vi "test Upload I32 C5-E.vi"(11 "Test Case In":refnum<class "Tests SDO Manager.lvclass">) -> (0 "error out":errorcluster, 3 "Test Case Out":refnum<class "Tests SDO Manager.lvclass">)   [LabVIEW 2020, in "Tests SDO Manager.lvclass"]
uses:
  Tests SDO Manager.lvclass
  C:/Program Files/National Instruments/LabVIEW 2026/vi.lib/Astemes/LUnit/Test Case.lvclass
  source/Logging/Logger/Logger.lvclass
  C:/Program Files/National Instruments/LabVIEW 2026/vi.lib/ActorFramework/Actor/Actor.lvclass
  HAL/HAL-Devices/source/PCAN USB Dongle/PCAN Basic 4/Configure Strategies/Read-Write CAN Frame Strategy/PCAN Basic4 Read-Write CAN CC Frame Strategy.lvclass
  D:/git/HAL/Source/Interfaces/IApplyConfiguration/IApplyConfiguration.lvclass
  HAL/Source/Communicator/Communicator.lvclass
  D:/git/HAL/Source/Interfaces/ICommunicate/ICommunicate.lvclass
  source/Logging/Logger/Logger.lvclass/Logger.ctl
  source/SDO Manager/SDO Manager/SDO Manager/SDO Manager.lvclass/SDO Manager.ctl
  <vilib>/ActorFramework/Message Enqueuer/Message Enqueuer.lvclass/Message Enqueuer.ctl
  <vilib>/Astemes/LUnit/Test Case.lvclass/Test Case.ctl
  <vilib>/ActorFramework/Stop Msg/Stop Msg.lvclass
  C:/Program Files/National Instruments/LabVIEW 2026/vi.lib/ActorFramework/Message/Message.lvclass
  HAL/Source/Interfaces/IMessage/IMessage.lvclass
  Tests SDO Manager.lvclass/Tests SDO Manager.ctl
  D:/git/HAL/HAL-Devices/source/PCAN USB Dongle/PCAN Basic 4/Configure Strategies/Base Configure Strategy/PCAN Basic4 Base Configure Strategy.lvclass
  D:/git/HAL/Source/Interfaces/IClose/IClose.lvclass
  D:/git/HAL/Source/Interfaces/IInitialize/IInitialize.lvclass
  D:/git/HAL/Source/Interfaces/IRunnable/IRunnable.lvclass
  D:/git/HAL/Source/Interfaces/IValidate Configuration/IValidate Configuration.lvclass
  D:/git/HAL/HAL-Devices/source/PCAN USB Dongle/PCAN Basic 4/Configure Strategies/Read-Write CAN Frame Strategy/PCAN Basic4 Read-Write CAN CC Frame Strategy.lvclass
  D:/git/HAL/Source/Interfaces/IInstrument/IInstrument.lvclass
  D:/git/HAL/Source/Communicator/Communicator.lvclass
  D:/git/HAL/Source/Interfaces/IConfigurable/IConfigurable.lvclass
  D:/git/CANopen-LabVIEW/source/Logging/Logger/Logger.lvclass
  4993e8ee-a06a-463a-9684-69129f64d5ce.vi
  source/SDO Manager/SDO Manager/SDO Manager/SDO Manager.lvclass
  source/Logging/Log Level.vi
  source/Logging/CANopen Logging.lvlib
  <vilib>/ActorFramework/Actor/Actor.lvclass
  source/SDO Manager/SDO Manager/SDO Manager/Upload I32.vi
  source/SDO Manager/SDO Manager/SDO Transfer/SDO abort code.ctl
  source/SDO Manager/SDO Manager/SDO Transfer/SDO Transfer.lvclass
  source/Typedefs/SDO Result.ctl
panel:
  out "SDO Result":T1={"Success"=FALSE, "SDO abort code"={"Null"=TRUE, "Value"=84082688}, "Data"={"Null"=TRUE, "Data"=[]}} {"SDO abort code"."Value" items=["Toggle bit not allowed"=84082688, "SDO protocol timed out"=84148224, "Client/server command specifier not valid or unknown"=84148225, "Invalid block size (block mode only)"=84148226, "Invalid sequence number (block mode only)"=84148227, "CRC error (block mode only)"=84148228, "Out of memory"=84148229, "Attempt to read a write only object"=100728833, "Attempt to write a read only object"=100728834, "Object does not exist in the object dictionary"=100794368, "Object cannot be mapped to the PDO"=100925505, "The number and length of the objects to be mapped would exceed PDO length"=100925506, "General parameter incompatibility reason"=100925507, "General internal incompatibility in the device"=100925511, "Access failed due to an hardware error"=101056512, "Data type does not match, length of service parameter does not match"=101122064, "Data type does not match, length of service parameter too high"=101122066, "Data type does not match, length of service parameter too low"=101122067, "Sub-index does not exist"=101253137, "Invalid value for parameter (download only)"=101253168, "Value of parameter written too high (download only)"=101253169, "Value of parameter written too low (download only)"=101253170, "Maximum value is less than minimum value"=101253174, "Resource not available: SDO connection"=101318691, "General error"=134217728, "Data cannot be transferred or stored to the application"=134217760, "Data cannot be transferred or stored to the application because of local control"=134217761, "Data cannot be transferred or stored to the application because of the present device stable"=134217762, "Object dictionary dynamic generation fails or no object dictionary is present (e.g. object dictionary is generated from file and generation fails because of an file error)"=134217763, "No data available"=134217764]; "Data"."Data" format="%02x"}
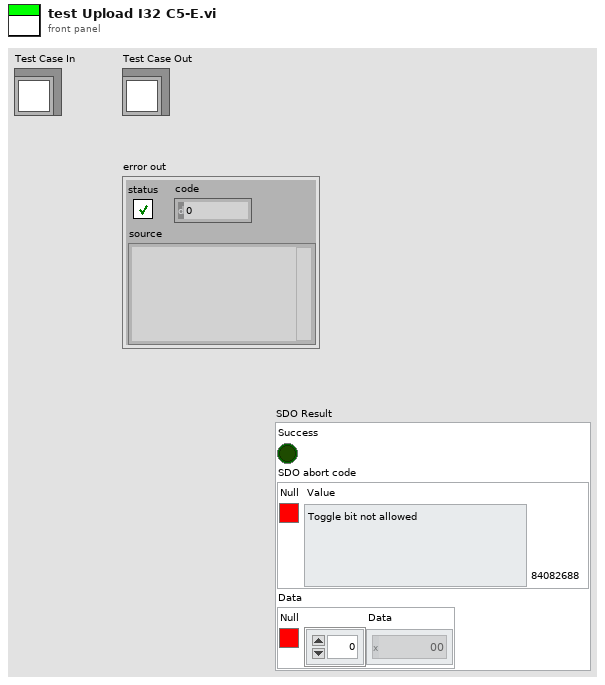
[diagram p1: front panel]
types:
  T1 = typedef "CANopen.lvlib/SDO Manager.lvlib/SDO Transfer.lvclass/SDO Result.ctl" = cluster{"Success":bool, "SDO abort code":cluster{"Null":bool, "Value":T2}, "Data":cluster{"Null":bool, "Data":u8[]}}
  T2 = typedef "CANopen.lvlib/SDO Manager.lvlib/SDO Transfer.lvclass/SDO abort code.ctl" = u32
  T3 = cluster{"Node-ID":u8, "Multiplexer":cluster{"Index":u16, "Sub-Index":u8}}
  T4 = enum16{"Error", "Warn", "Info", "Debug", "Trace"}
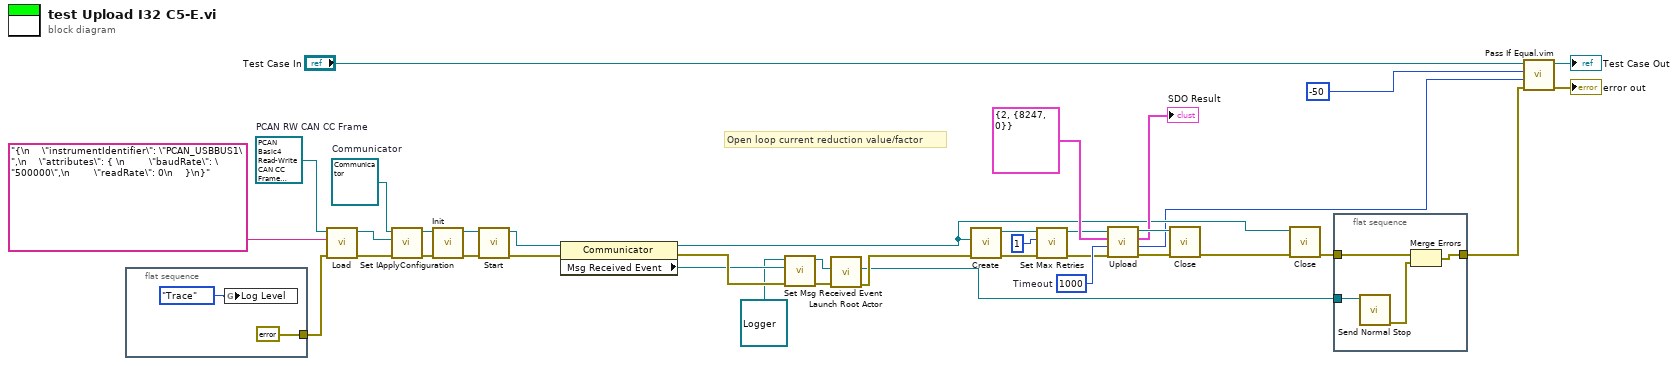
[diagram p0: block diagram]
diagram:
  w8 = refnum<class "Communicator.lvclass"> refnum  # Communicator
  w14 = refnum<class "PCAN Basic4 Read-Write CAN CC Frame Strategy.lvclass"> refnum  # PCAN RW CAN CC Frame
  w31 = 1000  # Timeout
  # "Open loop current reduction value/factor"
  n1 = flat-sequence {
    tunnel: [errorcluster {"status"=FALSE, "code"=0, "source"=""} ("error constant")] -> w3
    frame #0 {
      n2 = global write "Log Level.vi" "Log Level"(T4."Trace" ("Log Level")) -> ()
    }
  }
  n3 = call-dynamic "Load.vi"("error in"=w3, "Source"="{\n    \"instrumentIdentifier\": \"PCAN_USBBUS1\",\n    \"attributes\": { \n        \"baudRate\": \"500000\",\n        \"readRate\": 0\n    }\n}", "PCAN Basic Base Configure Strategy in"=w14) -> ("error out"=w11:errorcluster, "PCAN Basic Base Configure Strategy out"=w12:refnum<class "PCAN Basic4 Read-Write CAN CC Frame Strategy.lvclass">)  [unwired: 7 in]
  n4 = call-dynamic "Set IApplyConfiguration.vi"("Error In"=w11, "IApplyConfiguration"=w12, "Communicator in"=w8) -> ("Error Out"=w10:errorcluster, "Communicator out"=w9:refnum<class "Communicator.lvclass">)  [unwired: 7 in]
  n5 = call-dynamic "Init.vi"("Error In"=w10, "Communicator in"=w9) -> ("Error Out"=w7:errorcluster, "Communicator out"=w6:refnum<class "Communicator.lvclass">)  [unwired: 8 in]
  n6 = call-dynamic "Start.vi"("Error In"=w7, "Communicator in"=w6) -> ("Error Out"=w5:errorcluster, "Communicator out"=w4:refnum<class "Communicator.lvclass">)  [unwired: 8 in]
  n7 = property class="Communicator"(reference=w4, error in=w5) -> (reference out=w15:refnum<class "Communicator.lvclass">, error out=w27:errorcluster, "Msg Received Event"=w26:refnum<user-event>)
  n8 = call "Set Msg Received Event.vi"("error in"=w27, "Msg Received Event"=w26, "Logger in"=refnum<class "Logger.lvclass"> refnum) -> ("error out"=w29:errorcluster, "Logger out"=w28:refnum<class "Logger.lvclass">)  [unwired: 7 in]
  n9 = call <vilib>:"Launch Root Actor.vi"("error in (no error)"=w29, "Actor"=w28) -> ("error out"=w25:errorcluster, "Actor's Enqueuer"=w22:refnum<class "Message Enqueuer.lvclass">)  [unwired: 8 in]
  n10 = call "Create.vi"("Error In"=w25, "ICommunicate"=w15) -> ("Error Out"=w20:errorcluster, "SDO Manager"=w19:refnum<class "SDO Manager.lvclass">)  [unwired: 8 in]
  n11 = call "Set Max Retries.vi"("error in"=w20, "Max Retries"=u8 1, "SDO Manager in"=w19) -> ("error out"=w17:errorcluster, "SDO Manager out"=w18:refnum<class "SDO Manager.lvclass">)  [unwired: 7 in]
  n12 = call-poly "Upload.vi"("Error In"=w17, "Retry Delay (ms)"=w31, "Parameters"=T3 {"Node-ID"=2, "Multiplexer"={"Index"=8247, "Sub-Index"=0}}, "SDO Manager in"=w18) -> ("Error Out"=w33:errorcluster, "Value"=w1:i32, "SDO Result"=→"SDO Result":T1, "SDO Manager out"=w32:refnum<class "SDO Manager.lvclass">)  [unwired: 4 in]
  n13 = call "Close.vi"("Error In"=w33, "SDO Manager"=w32) -> ("Error Out"=w35:errorcluster)  [unwired: 8 in, 1 out]
  n14 = call-dynamic "Close.vi"("Error In"=w35, "Communicator in"=w15) -> ("Error Out"=w23:errorcluster)  [unwired: 8 in, 1 out]
  n15 = flat-sequence {
    tunnel: w23 -> [w41]
    tunnel: w22 -> [w44]
    tunnel: [w42] -> w21
    frame #0 {
      n16 = call <vilib>:"Send Normal Stop.vi"("Message Enqueuer"=w44) -> ("error out"=w43:errorcluster)  [unwired: 10 in]
      n17 = Merge Errors(w41, w43) -> (w42:errorcluster)
    }
  }
  n18 = call "Pass If Equal.vim"("error in (no error)"=w21, "Actual"=w1, "Expected"=-50, "LUnit Test Case In"="Test Case In") -> ("error out"=→"error out":errorcluster, "LUnit Test Case Out"=→"Test Case Out":refnum<class "Tests SDO Manager.lvclass">)  [unwired: 6 in]
